vi "Front-load.vi"(5 "Show UI?(F)":bool, 7 "Load Interrupt":refnum<notifier>, 8 "error in (no error)":errorcluster, 11 "Scope(Paths)":T1) -> (0 "error out":errorcluster, 1 "Success?":bool)   [LabVIEW 2020, in "ClassLoader.lvlib"]
uses:
  ClassLoader.lvlib
  Sub/Ctl/Ctl_Front-load Scope.ctl
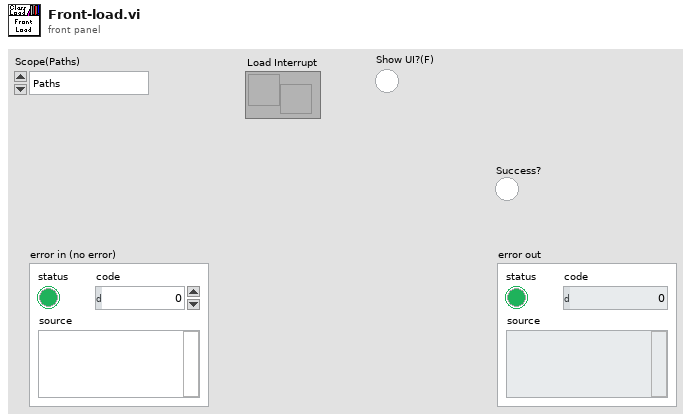
[diagram p1: front panel]
types:
  T1 = typedef "ClassLoader.lvlib/Ctl_Front-load Scope.ctl" = enum16{"Paths", "Paths and Hierarchies", "All"}
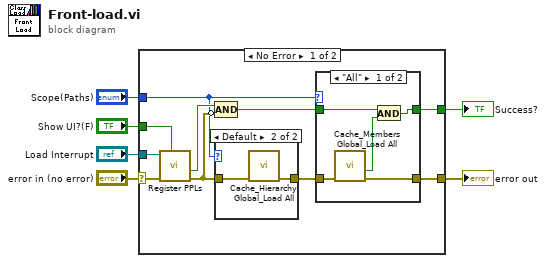
[diagram p0: block diagram]
diagram:
  n1 = case shown="No Error" "error in (no error)" {
    selector: "error in (no error)" -> [w16 w27]
    tunnel: [w10 w27] -> w5
    tunnel: [w8 _] -> w4
    tunnel: "Show UI?(F)" -> [w14 _]
    tunnel: "Load Interrupt" -> [w13 _]
    tunnel: "Scope(Paths)" -> [w9 _]
    frame No Error {
      n2 = call "Register PPLs.vi"("Show UI?(F)"=w14, "error in"=w16, "Interrupt"=w13) -> ("error out"=w12:errorcluster, "Success?"=w15:bool)  [unwired: 7 in]
      n3 = Compound Arithmetic op=AND(w15, invert w12) -> (w7:bool)
      n4 = case shown="Default" w9 {
        tunnel: [w24 w26] -> w11
        tunnel: w12 -> [w24 w25]
        frame "Paths" {
        }
        frame Default {
          n5 = call "Cache_Hierarchy Global_Load All.vi"("error in (no error)"=w25) -> ("error out"=w26:errorcluster)  [unwired: 9 in, 1 out]
        }
      }
      n6 = case shown="\"All\"" w9 {
        tunnel: [w21 w23] -> w10
        tunnel: w11 -> [w20 w23]
        tunnel: [w17 w22] -> w8
        tunnel: w7 -> [w19 w22]
        frame "All" {
          n7 = call "Cache_Members Global_Load All.vi"("error in (no error)"=w20) -> ("error out"=w21:errorcluster, "All Success?"=w18:bool)  [unwired: 8 in, 1 out]
          n8 = And(x=w19, y=w18) -> (x .and. y?=w17:bool)
        }
        frame Default {
        }
      }
    }
    frame Error {
    }
  }
  "error out" <- w5
  "Success?" <- w4
